vi "miguelzin do grau 04.02.vi"() -> (0 "timestamp":dbl[](array[numeric]), 1 "C":dbl[](graph), 2 "B":dbl[](graph), 3 "A":dbl[](graph))   [LabVIEW 2024]
uses:
  <vilib>/numeric/Random Number (Range) DBL.vi
panel:
  out "Potencial Ativa C":dbl[](array[numeric])
  out "Tensão C":dbl[](array[numeric])
  out "Corrente C":dbl[](array[numeric])
  out "FP 3":dbl
  in  "Limite Superior - FP  2":dbl=100.0
  in  "Limite Inferior - FP 3":dbl
  out "Potencial Ativa B":dbl[](array[numeric])
  out "Tensão B":dbl[](array[numeric])
  out "Corrente B":dbl[](array[numeric])
  out "FP 2":dbl
  in  "Limite Superior - FP":dbl=100.0
  in  "Limite Inferior - FP 2":dbl
  out "Potencial Ativa A":dbl[](array[numeric])
  out "Tensão A":dbl[](array[numeric])
  out "Corrente A":dbl[](array[numeric])
  out "FP":dbl
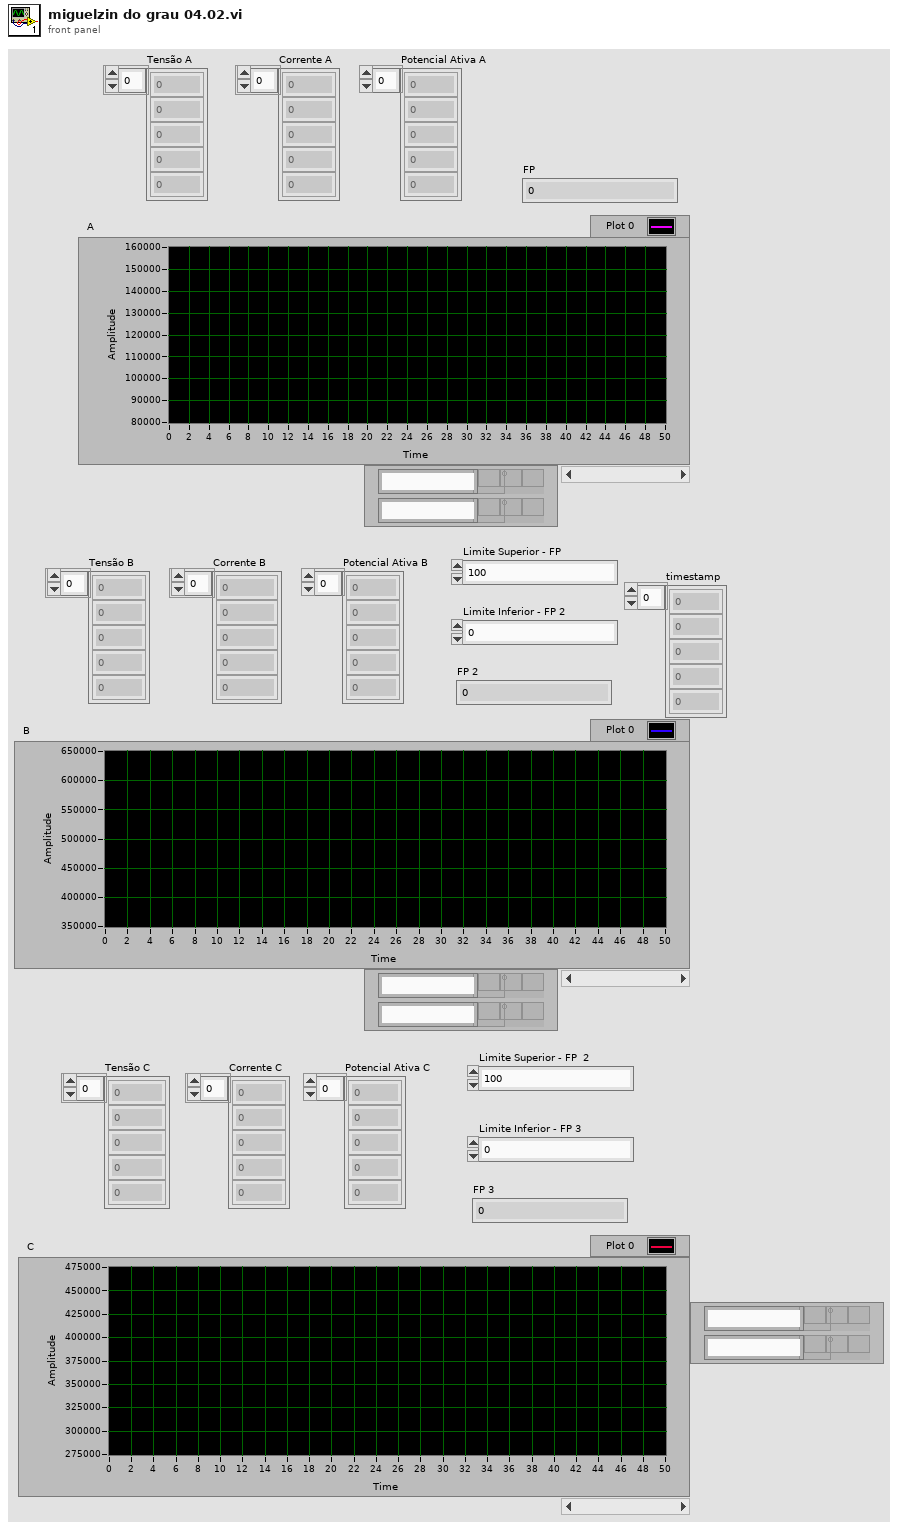
[diagram p1: front panel]
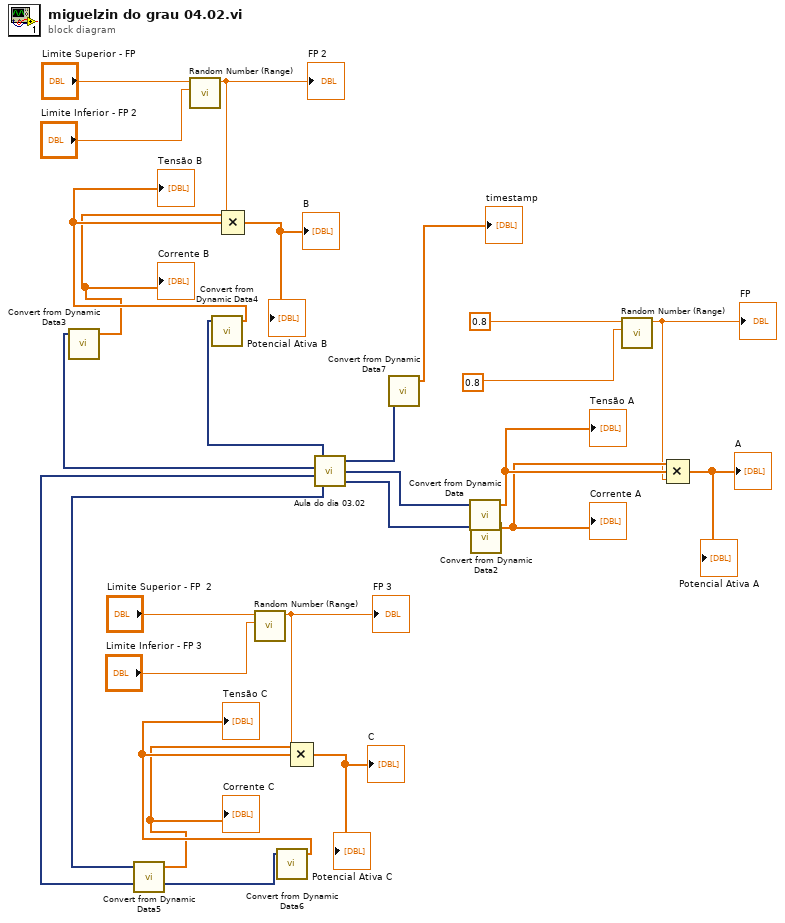
[diagram p0: block diagram]
diagram:
  n1 = call-poly <vilib>:"Random Number (Range).vi"("lower bound (0)"="Limite Inferior - FP 2", "upper bound (100)"="Limite Superior - FP") -> ("number"=w16:dbl)  [unwired: 9 in]
  "FP 2" <- w16
  n2 = call-poly <vilib>:"Random Number (Range).vi"("lower bound (0)"="Limite Inferior - FP 3", "upper bound (100)"="Limite Superior - FP  2") -> ("number"=w10:dbl)  [unwired: 9 in]
  "FP 3" <- w10
  n3 = call "Aula do dia 03.02.vi"() -> ("Corrente Fase A"=w26:dynamicdata, "Tensão Fase A"=w25:dynamicdata, "Timestamp"=w4:dynamicdata, "Corrente Fase C"=w6:dynamicdata, "Tensão Fase C"=w5:dynamicdata, "Corrente Fase B"=w19:dynamicdata, "Tensão Fase B"=w20:dynamicdata)
  n4 = call "Convert from Dynamic Data3"("Dynamic Data Type"=w19) -> ("Array"=w13:dbl[])  [unwired: 3 in]
  "Corrente B" <- w13
  n5 = call "Convert from Dynamic Data5"("Dynamic Data Type"=w6) -> ("Array"=w7:dbl[])  [unwired: 3 in]
  "Corrente C" <- w7
  n6 = call "Convert from Dynamic Data4"("Dynamic Data Type"=w20) -> ("Array"=w14:dbl[])  [unwired: 3 in]
  "Tensão B" <- w14
  n7 = Compound Arithmetic op=MULTIPLY(w13, w14, w16) -> (→"B" →"Potencial Ativa B":dbl[])
  n8 = call "Convert from Dynamic Data6"("Dynamic Data Type"=w5) -> ("Array"=w8:dbl[])  [unwired: 3 in]
  "Tensão C" <- w8
  n9 = Compound Arithmetic op=MULTIPLY(w7, w8, w10) -> (→"C" →"Potencial Ativa C":dbl[])
  n10 = call "Convert from Dynamic Data7"("Dynamic Data Type"=w4) -> ("Array"=→"timestamp":dbl[])  [unwired: 3 in]
  n11 = call "Convert from Dynamic Data"("Dynamic Data Type"=w25) -> ("Array"=w24:dbl[])  [unwired: 3 in]
  "Tensão A" <- w24
  n12 = call "Convert from Dynamic Data2"("Dynamic Data Type"=w26) -> ("Array"=w23:dbl[])  [unwired: 3 in]
  "Corrente A" <- w23
  n13 = call-poly <vilib>:"Random Number (Range).vi"("lower bound (0)"=0.8, "upper bound (100)"=0.8) -> ("number"=w22:dbl)  [unwired: 9 in]
  "FP" <- w22
  n14 = Compound Arithmetic op=MULTIPLY(w23, w24, w22) -> (→"A" →"Potencial Ativa A":dbl[])
